vi "test_TxGen-RxMon.vi"(8 "error in":errorcluster, 11 "reference in":refnum<class "AIM ARINC 664 Loopback.lvclass">) -> (0 "error out":errorcluster, 3 "reference out":refnum<class "AIM ARINC 664 Loopback.lvclass">)   [LabVIEW 2020, in "AIM ARINC 664 Loopback.lvclass"]
uses:
  AIM ARINC 664 Loopback.lvclass
  C:/Program Files (x86)/National Instruments/LabVIEW 2020/vi.lib/addons/_JKI Toolkits/VI Tester/TestCase.llb/TestCase.lvclass
  AIM ARINC 664 Loopback.lvclass/AIM ARINC 664 Loopback.ctl
  <vilib>/addons/_JKI Toolkits/VI Tester/TestCase.llb/TestCase.lvclass
  <vilib>/NI VeriStand/Execution/Workspace/NI_VS Workspace ExecutionAPI.lvlib
  6a3dd3ed-914d-4d14-bf18-724521aa5e28.vi
  NationalInstruments.VeriStand.SystemDefinitionAPI
  Scripting/AIM ARINC 664 Scripting.lvlib
  Import/AIM ARINC 664 Import.lvlib
  56c9d474-e1ad-41d5-9732-7ebb07e8a0f2.vi
  3f9c4eda-19e9-4962-b6bc-794414341bbb.vi
  <vilib>/NI VeriStand/Execution/Workspace/NI VeriStand - Get Multiple Channel Values.vi
  C:/Program Files/National Instruments/LabVIEW 2024/vi.lib/addons/_JKI Toolkits/VI Tester/TestCase.llb/TestCase.lvclass
panel:
  out "Elapsed Time (s)":dbl
  out "Values":dbl[](array[numeric])
  in  "tolerance (5 samples)":dbl=20.0 caption="Time Target (s)"
  in  "Time Target (s)":dbl=5.0
  # "This test is disabled fro now because the configuration is between two cards. If \nyou need to setup this, change from the two cards to one card configuration as below:"
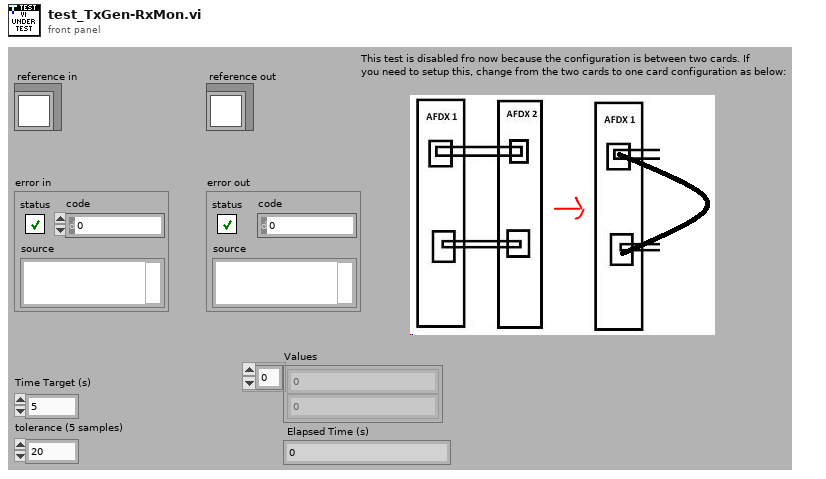
[diagram p1: front panel]
types:
  T1 = typedef "Custom Device API.lvlib/Custom Device Item Ref.ctl" = u64
  T2 = typedef "AIM ARINC 664 Import.lvlib/Board Top Level Configuration.ctl" = cluster{"boardSetup":T3, "portConfiguration":T4[]}
  T3 = typedef "AIM ARINC 664 Import.lvlib/board_setup.ctl" = cluster{"boardId":u32, "portSpeed":u32, "portConfig":u32}
  T4 = typedef "AIM ARINC 664 Import.lvlib/port_configuration.ctl" = cluster{"portSetup":T5, "Tx_Generic":T6[], "Rx_Monitor":cluster{"DefaultCronoMode":u32, "GlbMonBufferSizeIn":u32, "CaptureMode":u32, "MaxFileSizeMB":u32, "Strobe":u32, "TriggerPosition":u32}[], "Tx_UDP":cluster{"tx_udp_setup":cluster{"VlId":i32, "Bag":i32, "NetSelect":u32, "domainID":u8, "sideID":u8, "locationID":u8, "interfaceID":u8, "NumOfSubVl":u16, "Skew":u32, "MaxFrameLength":u32, "FrameBufferSize":u32}, "commPorts":T14[], "sapPorts":T15[]}[], "Rx_UDP":cluster{"Tx_UDP":T16, "commPorts":T17[], "sapPorts":T18[]}[]}
  T5 = typedef "AIM ARINC 664 Import.lvlib/port_setup.ctl" = cluster{"port Id":u32, "redundant":bool}
  T6 = typedef "AIM ARINC 664 Import.lvlib/session_tx_generic.ctl" = cluster{"tx_generic_setup":T7, "Frame Headers":T8[]}
  T7 = typedef "AIM ARINC 664 Import.lvlib/tx_generic_setup.ctl" = cluster{"QueueSizeIn":u32, "Count":i32, "StartMode":i32}
  T8 = typedef "AIM ARINC 664 Import.lvlib/frame_tx_generic.ctl" = cluster{"FrameID":string, "PayloadID":string, "Frame header":cluster{"FrameStartMode":i32, "InterFrameGap":i32, "PacketGroupWaitTime":i32, "NetSelect":u32, "PayloadBufferMode":i32, "PayloadGenerationMode":i32, "PhysErrorInjection":i32, "PreambleCount":i32, "SequenceNumberInit":T9, "SequenceNumberOffset":T10, "Skew":i32}, "Parameters":T11[]}
  T9 = typedef "AIM ARINC 664 Import.lvlib/frame_tx_generic_seqNumberInit.ctl" = i32
  T10 = typedef "AIM ARINC 664 Import.lvlib/frame_tx_generic_seqNumberOffset.ctl" = i32
  T11 = typedef "AIM ARINC 664 Import.lvlib/frame_parameter.ctl" = cluster{"name":string, "default value":dbl, "unit":string, "Parameter":T12}
  T12 = typedef "AIM ARINC 664 Import.lvlib/frame_parameter_definition.ctl" = cluster{"start index":i32, "size":i32, "encoding":T13, "signed":bool, "scale multiplier":dbl, "scale offset":dbl}
  T13 = typedef "Encoding (Arinc664).ctl" = u16
  T14 = typedef "AIM ARINC 664 Import.lvlib/port_tx_udp_comm.ctl" = cluster{"PayloadID":string, "partitionID":u8, "UdpSrcPort":u16, "UdpDstPort":u16, "PortType":enum16{"FDX_UDP_SAMPLING", "FDX_UDP_QUEUING"}, "SubVIId":u32, "UdpNumBufMessages":u32, "UdpMaxMessageSize":u32, "UdpSamplingRate":u32, "Parameters":T11[]}
  T15 = typedef "AIM ARINC 664 Import.lvlib/port_tx_udp_sap.ctl" = cluster{"PayloadID":string, "SubVlId":u8, "UdpSrcPort":u16, "UdpNumBufMessages":u32, "UdpMaxMessageSize":u32, "partitionID":u8, "domainID":u8, "sideID":u8, "locationID":u8, "interfaceID":u8, "Parameters":T11[]}
  T16 = typedef "AIM ARINC 664 Import.lvlib/rx_udp_setup.ctl" = cluster{"VerificationMode":u32, "Bag":u32, "Jitter":u32, "MaxFrameLength":u32, "MaxSkew":u32, "VLBufSize":u32, "FilterMode":u32, "FilterPosition":u32, "Padding":u32, "FilterMask":u32, "FilterData":u32, "MinFrameLength":u32, "VlId":u16, "VLRange":u32}
  T17 = typedef "AIM ARINC 664 Import.lvlib/port_rx_udp_comm.ctl" = cluster{"PayloadID":string, "domainID":u8, "sideID":u8, "locationID":u8, "partitionID":u8, "UdpSrcPort":u16, "UdpDstPort":u16, "PortType":enum16{"FDX_UDP_SAMPLING", "FDX_UDP_QUEUING"}, "SubVIId":u32, "UdpNumBufMessages":u32, "UdpMaxMessageSize":u32, "UdpSamplingRate":u32, "Parameters":T11[]}
  T18 = typedef "AIM ARINC 664 Import.lvlib/port_rx_udp_sap.ctl" = cluster{"PayloadID":string, "UdpDstPort":u16, "UdpNumBufMessages":u32, "UdpMaxMessageSize":u32, "Parameters":T11[]}
  T19 = typedef "Payload Map.ctl" = map{string, T20}
  T20 = typedef "Payload Record Type.ctl" = cluster{"Data":u8[], "Type of Frame":T21}
  T21 = typedef "Type of Payload.ctl" = u16
  T22 = typedef "NI_VS Workspace ExecutionAPI.lvlib/WorkspaceAPI.ctl" = refnum<k24>
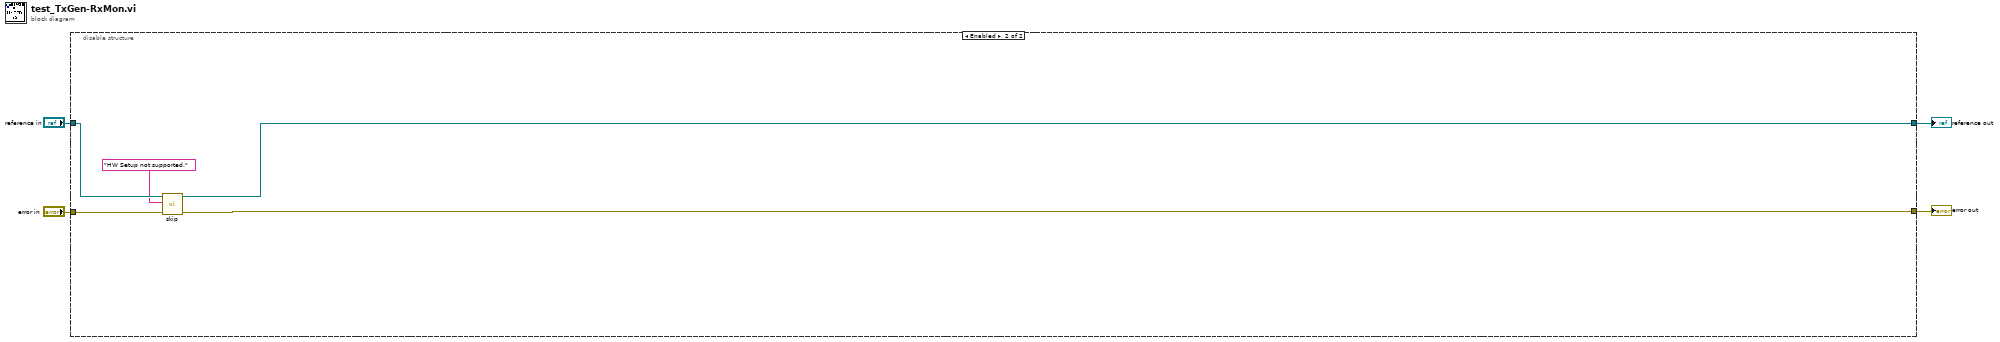
[diagram p0: block diagram]
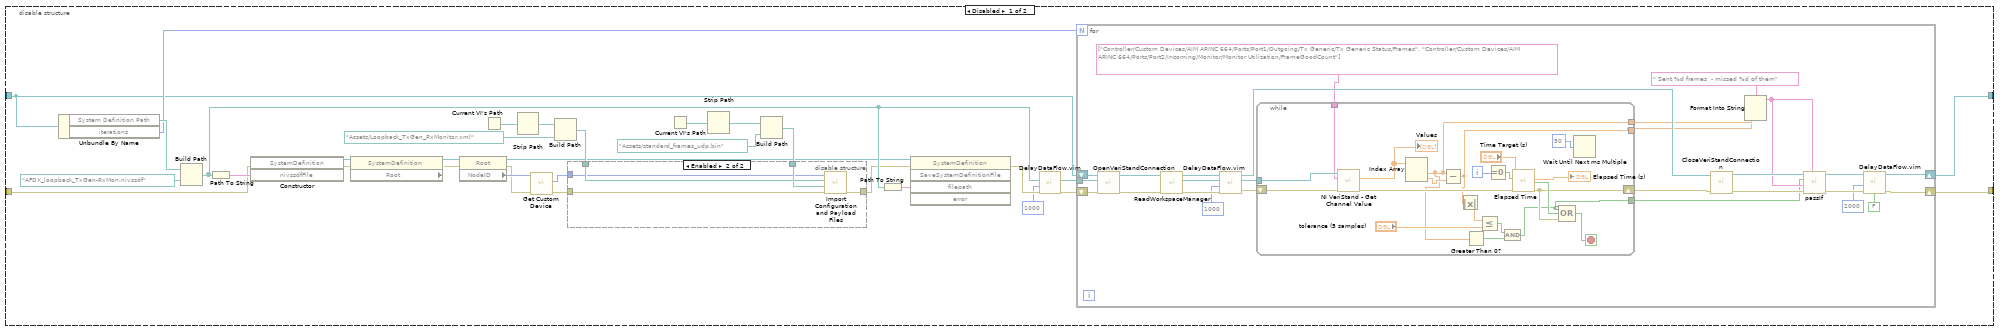
[diagram p2: hidden frame]
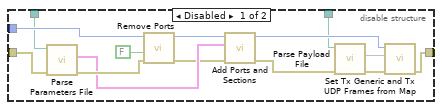
[diagram p3: hidden frame]
diagram:
  n1 = disable-structure shown="Enabled" {
    disable-tunnel: "reference in" -> [w5 w104]
    disable-tunnel: "error in" -> [w6 w103]
    disable-tunnel: [w35 w102] -> w2
    disable-tunnel: [w34 w101] -> w1
    frame Disabled {
      n2 = Unbundle By Name(w5) -> ("System Definition Path"=w33:path, "iterations"=w11:i32)
      n3 = Build Path(base path=w33, name or relative path=path "AFDX_loopback_TxGen-RxMon.nivssdf") -> (appended path=w30:path)
      n4 = Path To String(path=w30) -> (string=w31:string)
      n5 = constructor class="SystemDefinition"(error in=w6, "nivssdfFile"=w31) -> (reference out=w29:refnum<k24>, error out=w27:errorcluster)  [unwired: 2 in, 2 out]
      n6 = property class="SystemDefinition"(reference=w29, error in=w27) -> (reference out=w17:refnum<k24>, error out=w26:errorcluster, "Root"=w28:refnum<k24>)
      n7 = property class="Root"(reference=w28, error in=w26) -> (error out=w14:errorcluster, "NodeID"=w15:u64)  [unwired: 1 out]
      n8 = Current VI's Path() -> (path=w25:path)
      n9 = Strip Path(path=w25) -> (stripped path=w20:path)  [unwired: 1 out]
      n10 = call "Get Custom Device.vi"("error in"=w14, "custom device ref in"=w15) -> ("error out"=w13:errorcluster, "First Item Ref"=w12:T1)  [unwired: 5 in, 3 out]
      n11 = Build Path(base path=w20, name or relative path=path "Assets/Loopback_TxGen_RxMonitor.xml") -> (appended path=w21:path)
      n12 = Current VI's Path() -> (path=w24:path)
      n13 = Strip Path(path=w24) -> (stripped path=w19:path)  [unwired: 1 out]
      n14 = Build Path(base path=w19, name or relative path=path "Assets/standard_frames_udp.bin") -> (appended path=w22:path)
      n15 = disable-structure shown="Enabled" {
        disable-tunnel: w12 -> [w93 w95]
        disable-tunnel: w13 -> [w85 w99]
        disable-tunnel: w22 -> [w83 w96]
        disable-tunnel: w21 -> [w82 w97]
        disable-tunnel: [w81 w98] -> w18
        frame Disabled {
          n16 = call "Parse Parameters File.vi"("error in"=w85, "path to XML document"=w82) -> ("error out"=w94:errorcluster, "board configuration out"=w91:T2)  [unwired: 7 in, 1 out]
          n17 = call "Remove Ports.vi"("error in"=w94, "refresh?"=FALSE, "Custom device Ref"=w93) -> ("error out"=w90:errorcluster, "Custom device Ref out"=w92:T1)  [unwired: 7 in]
          n18 = call "Add Ports and Sections.vi"("error in"=w90, "board configuration in"=w91, "custom device ref"=w92) -> ("error out"=w89:errorcluster, "custom device ref out"=w84:T1)  [unwired: 7 in]
          n19 = call "Parse Payload File.vi"("error in"=w89, "frame array path in"=w83) -> ("error out"=w88:errorcluster, "Map"=w87:T19)  [unwired: 7 in, 1 out]
          n20 = call "Set Tx Generic and Tx UDP Frames from Map.vi"("error in"=w88, "payload map"=w87, "custom device ref"=w84) -> ("error out"=w81:errorcluster)  [unwired: 7 in, 1 out]
        }
        frame Enabled {
          n21 = call "Import Configuration and Payload Files.vi"("error in"=w99, "payload file path"=w96, "parameters configuration file path"=w97, "custom device ref"=w95) -> ("error out"=w98:errorcluster)  [unwired: 6 in, 1 out]
        }
      }
      n22 = Path To String(path=w30) -> (string=w16:string)
      n23 = invoke class="SystemDefinition" method="SaveSystemDefinitionFile"(reference=w17, error in=w18, "filepath"=w16) -> (error out=w9:errorcluster)  [unwired: 2 in, 4 out]
      n24 = call "DelayDataFlow.vim"("value in"=w9, "milliseconds to wait"=u32 1000) -> ("value out"=w8:errorcluster)  [unwired: 2 in, 1 out]
      n25 = for {
        N: w11 -> [_]
        tunnel: w30 -> [w41]
        shift-right: [w58] -> w34
        shift-left: w5 -> [w59]
        shift-right: [w39] -> w35
        shift-left: w8 -> [w42]
        n26 = call-dynamic "OpenVeriStandConnection.vi"("error in (no error)"=w42, "System Definition File"=w41, "VeriStand Test Case in"=w59) -> ("error out"=w57:errorcluster, "VeriStand Test Case out"=w52:refnum<class "AIM ARINC 664 Loopback.lvclass">)  [unwired: 6 in, 1 out]
        n27 = call-dynamic "ReadWorkspaceManager.vi"("error in (no error)"=w57, "VeriStand Test Case in"=w52) -> ("error out"=w47:errorcluster, "Workspace"=w50:T22, "VeriStand Test Case out"=w51:refnum<class "AIM ARINC 664 Loopback.lvclass">)  [unwired: 7 in]
        n28 = call "DelayDataFlow.vim"("value in"=w47, "milliseconds to wait"=u32 1000) -> ("value out"=w46:errorcluster)  [unwired: 2 in, 1 out]
        n29 = while {
          tunnel: w50 -> [w80]
          shift-right: [w73] -> w49
          shift-left: w46 -> [w78]
          tunnel: [w66] -> w48
          tunnel: [w65] -> w44
          tunnel: [w64] -> w43
          tunnel: string[] ["Controller/Custom Devices/AIM ARINC 664/Ports/Port1/Outgoing/Tx Generic/Tx Generic Status/Frames", "Controller/Custom Devices/AIM ARINC 664/Ports/Port2/Incoming/Monitor/Monitor Utilization/FrameGoodCount"] ("Channels") -> [w62]
          i -> [w61]
          stop <- w75 stop-if-true
          n30 = call-poly <vilib>:"NI VeriStand - Get Channel Value.vi"("error in (no error)"=w78, "Channels"=w62, "WorkspaceManager in"=w80) -> ("error out"=w77:errorcluster, "Values"=w72:dbl[])  [unwired: 6 in, 1 out]
          "Values" <- w72
          n31 = Index Array(array=w72) -> (element #1=w65:dbl, element #2=w71:dbl)  [unwired: 2 in]
          n32 = Subtract(x=w65, y=w71) -> (x-y=w64:dbl)
          n33 = Absolute Value(x=w64) -> (abs(x)=w70:dbl)
          n34 = Greater Than 0?(x=w65) -> (x > 0?=w67:bool)
          n35 = Less Or Equal?(x=w70, y="tolerance (5 samples)") -> (x <= y?=w68:bool)
          n36 = Equal To 0?(x=w61) -> (x = 0?=w60:bool)
          n37 = And(x=w68, y=w67) -> (x .and. y?=w66:bool)
          n38 = call "Elapsed Time"("Time Target (s)"="Time Target (s)", "Reset"=w60, "error in (no error)"=w77) -> ("Elapsed Time (s)"=→"Elapsed Time (s)":dbl, "Time has Elapsed"=w76:bool, "error out"=w73:errorcluster)  [unwired: 9 in, 5 out]
          n39 = Compound Arithmetic op=OR(invert w66, w76, w73) -> (w75:bool)
          n40 = Wait Until Next ms Multiple(millisecond multiple=u32 50 ("millisecond timer value")) -> ()  [unwired: 1 out]
        }
        n41 = call-dynamic "CloseVeriStandConnection.vi"("error in (no error)"=w49, "VeriStand Test Case in"=w51) -> ("error out"=w56:errorcluster, "VeriStand Test Case out"=w55:refnum<class "AIM ARINC 664 Loopback.lvclass">)  [unwired: 8 in]
        n42 = Format Into String(format string=" Sent %d frames  - missed %d of them", w44, w43) -> (resulting string=w53:string)  [unwired: 2 in, 1 out]
        n43 = call-dynamic "passIf.vi"("custom report message (\"\")"=w53, "error in (no error)"=w56, "message (\"\")"=w53, "pass"=w48, "TestCase in"=w55) -> ("error out"=w38:errorcluster, "TestCase out"=w58:refnum<class "AIM ARINC 664 Loopback.lvclass">)  [unwired: 5 in]
        n44 = call "DelayDataFlow.vim"("value in"=w38, "milliseconds to wait"=u32 2000, "no delay on error (T)"=FALSE) -> ("value out"=w39:errorcluster)  [unwired: 1 in, 1 out]
      }
    }
    frame Enabled {
      n45 = call <vilib>:"skip.vi"("error in (no error)"=w103, "skipMessage"="HW Setup not supported.", "TestCase in"=w104) -> ("error out"=w102:errorcluster, "TestCase out"=w101:refnum<class "AIM ARINC 664 Loopback.lvclass">)  [unwired: 7 in]
    }
  }
  "error out" <- w2
  "reference out" <- w1
